vi "Module Init.vi"(8 "error in (no error)":errorcluster, 11 "System Config Server in":refnum<class "System Config Module.lvclass">) -> (0 "error out":errorcluster, 3 "System Config Server out":refnum<class "System Config Module.lvclass">)   [LabVIEW 2020, in "Volatus.lvlib" / "System Config Module.lvclass"]
uses:
  System Config Module.lvclass
  System Config Module.lvclass/System Config Module.ctl
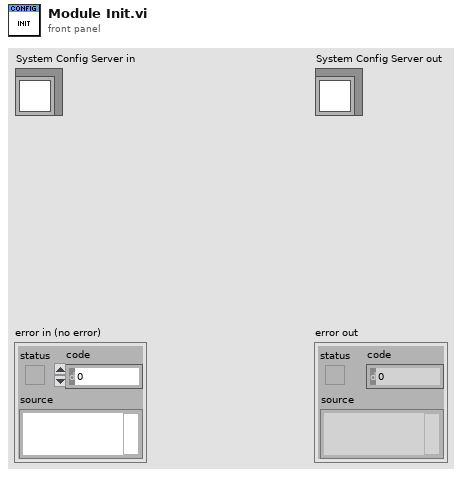
[diagram p1: front panel]
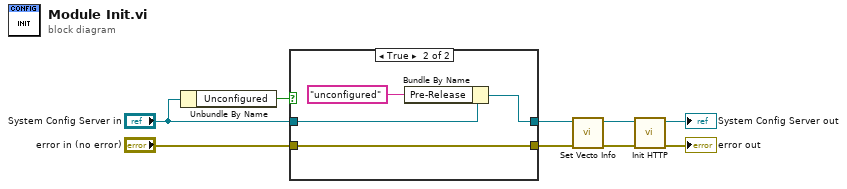
[diagram p0: block diagram]
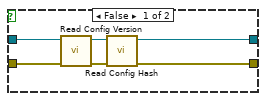
[diagram p2: hidden frame]
diagram:
  n1 = Unbundle By Name("System Config Server in") -> ("Unconfigured"=w1:bool)
  n2 = case shown="True" w1 {
    tunnel: "error in (no error)" -> [w13 w18]
    tunnel: [w12 w18] -> w8
    tunnel: [w11 w16] -> w4
    tunnel: "System Config Server in" -> [w10 w19]
    frame False {
      n3 = call "Read Config Version.vi"("error in (no error)"=w13, "System Config Server in"=w10) -> ("error out"=w14:errorcluster, "System Config Server out"=w15:refnum<class "System Config Module.lvclass">)  [unwired: 8 in]
      n4 = call "Read Config Hash.vi"("error in (no error)"=w14, "System Config Server in"=w15) -> ("error out"=w12:errorcluster, "System Config Server out"=w11:refnum<class "System Config Module.lvclass">)  [unwired: 8 in]
    }
    frame True {
      n5 = Bundle By Name(cluster=w19, "Pre-Release"="unconfigured") -> (w16:refnum<class "System Config Module.lvclass">)
    }
  }
  n6 = call "Set Vecto Info.vi"("error in (no error)"=w8, "System Config Module in"=w4) -> ("error out"=w5:errorcluster, "System Config Module out"=w3:refnum<class "System Config Module.lvclass">)  [unwired: 8 in]
  n7 = call "Init HTTP.vi"("error in (no error)"=w5, "System Config Server in"=w3) -> ("error out"=→"error out":errorcluster, "System Config Server out"=→"System Config Server out":refnum<class "System Config Module.lvclass">)  [unwired: 8 in]
